vi "VariablesToString_String.vi"(3 "Format":string, 4 "Terminate?":bool=TRUE, 5 "ValueIn":string, 6 "FieldName":string, 7 "Type":enum16{"Normal", "Matlab"}(ring)) -> (1 "StringOut":string)   [LabVIEW 2013]
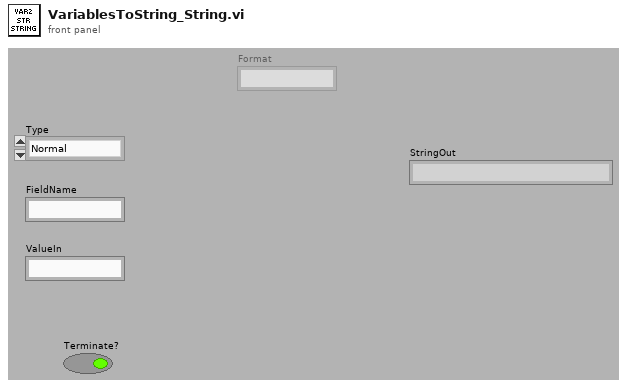
[diagram p1: front panel]
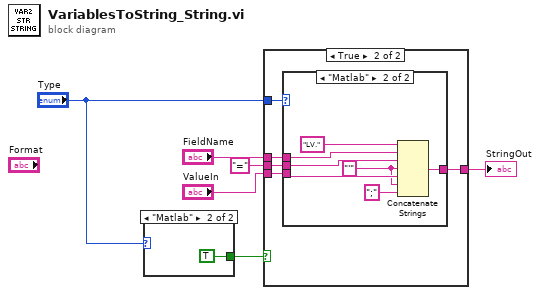
[diagram p0: block diagram]
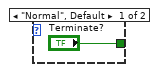
[diagram p2: hidden frame]
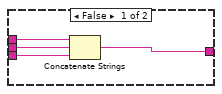
[diagram p3: hidden frame]
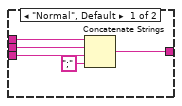
[diagram p4: hidden frame]
diagram:
  n1 = case shown="\"Matlab\"" "Type" {
    tunnel: ["Terminate?" TRUE ("Terminate?")] -> w3
    frame "Normal", Default {
    }
    frame "Matlab" {
    }
  }
  n2 = case shown="True" w3 {
    tunnel: "FieldName" -> [w12 w17]
    tunnel: "=" ("string") -> [w11 w16]
    tunnel: [w10 w15] -> w4
    tunnel: "ValueIn" -> [w9 w14]
    tunnel: "Type" -> [_ w13]
    frame False {
      n3 = Concatenate Strings(w12, w11, w9) -> (w10:string)
    }
    frame True {
      n4 = case shown="\"Matlab\"" w13 {
        tunnel: w17 -> [w22 w27]
        tunnel: w16 -> [w21 w26]
        tunnel: [w18 w29] -> w15
        tunnel: w14 -> [w20 w25]
        frame "Normal", Default {
          n5 = Concatenate Strings(w22, w21, w20, ";" ("string")) -> (w18:string)
        }
        frame "Matlab" {
          w24 = "'" ("string")
          n6 = Concatenate Strings("LV." ("string"), w27, w26, w24, w25, w24, ";" ("string")) -> (w29:string)
        }
      }
    }
  }
  "StringOut" <- w4
